vi "replace VI and XML GUIDs.vi"(8 "error in":errorcluster, 11 "custom device path":path=path "C:/Users/nitest/Documents/LabVIEW Data") -> (0 "error out":errorcluster, 3 "custom device path out":path=path "C:/Users/nitest/Documents/LabVIEW Data")   [LabVIEW 2020, in "Template Tool.lvlib"]
uses:
  Template Tool.lvlib
  Template Tool Global.vi
  GUID Tool/GUID Tool.lvlib
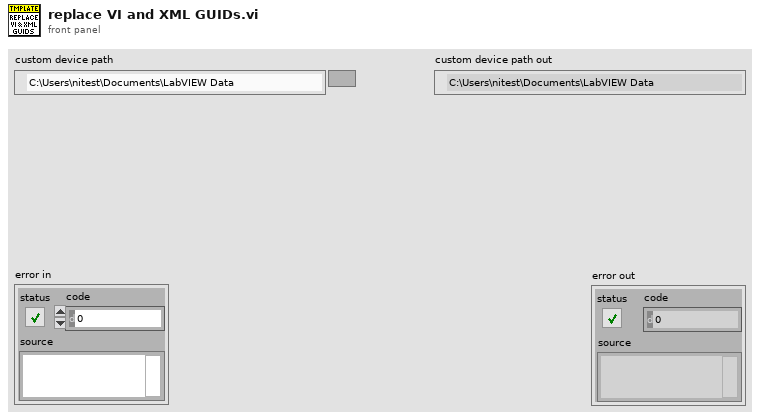
[diagram p1: front panel]
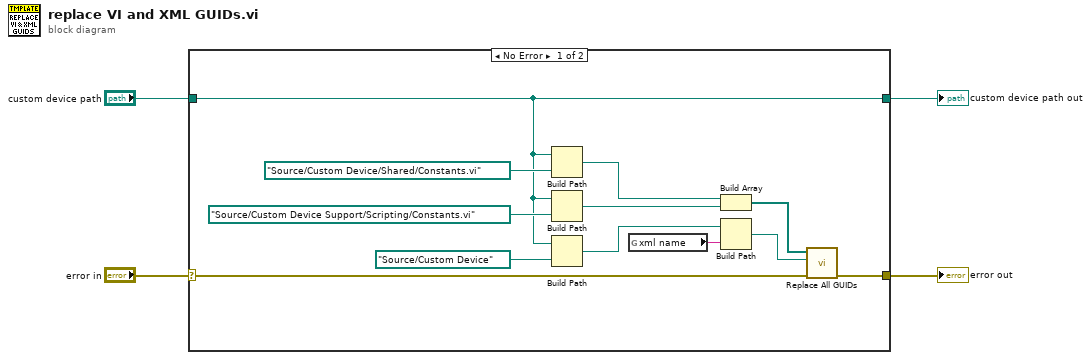
[diagram p0: block diagram]
diagram:
  n1 = case shown="No Error" "error in" {
    selector: "error in" -> [w10 w18]
    tunnel: [w8 w18] -> w4
    tunnel: "custom device path" -> [w9 w17]
    tunnel: [w9 w17] -> w1
    frame No Error {
      n2 = Build Path(base path=w9, name or relative path=path "Source/Custom Device/Shared/Constants.vi") -> (appended path=w14:path)
      n3 = Build Path(base path=w9, name or relative path=path "Source/Custom Device Support/Scripting/Constants.vi") -> (appended path=w13:path)
      n4 = Build Path(base path=w9, name or relative path=path "Source/Custom Device") -> (appended path=w11:path)
      n5 = global read "Template Tool Global.vi" "xml name"() -> (w5:string)
      n6 = Build Array(w14, w13) -> (w7:path[])
      n7 = Build Path(base path=w11, name or relative path=w5) -> (appended path=w6:path)
      n8 = call "Replace All GUIDs.vi"("error in"=w10, "xml path"=w6, "constants vi paths"=w7) -> ("error out"=w8:errorcluster)  [unwired: 8 in]
    }
    frame Error {
    }
  }
  "error out" <- w4
  "custom device path out" <- w1
